vi "CmdExe.Check StdOut, StdError, and Return Code for errors, Merge to Output Data.vi"(6 "Error Check":T1, 7 "App Name":string, 8 "error in":errorcluster, 9 "Return Code":i32, 10 "StdError":string, 11 "StdOut":string) -> (0 "error out":errorcluster, 3 "Output Data":string)   [LabVIEW 2024]
uses:
  CmdExe.Output Error Check Setup.ctl
  Errors/Error.Error Code List.ctl
  <vilib>/Utility/error.llb/Trim Whitespace One-Sided.vi
  Errors.lvlib
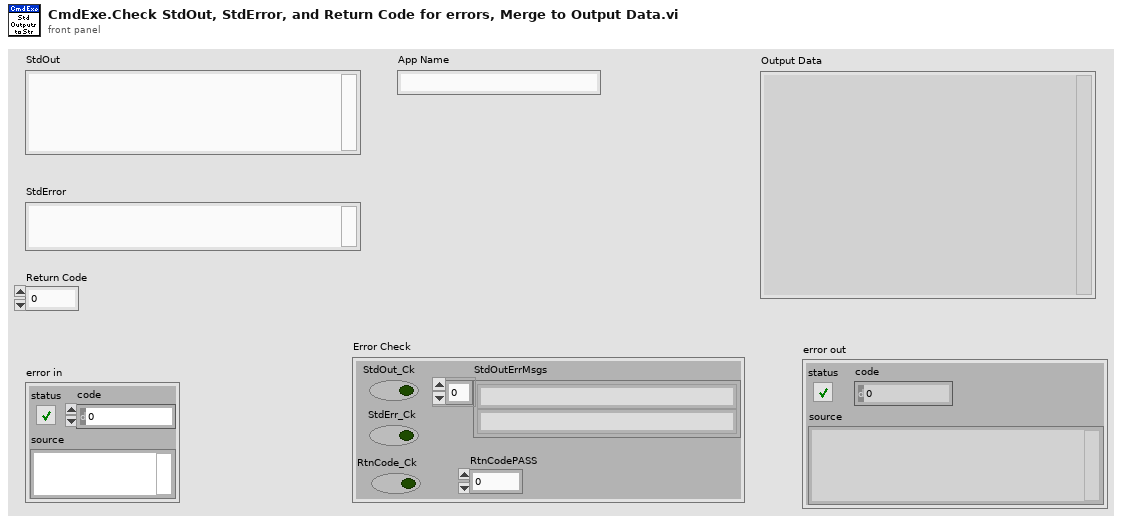
[diagram p1: front panel]
types:
  T1 = typedef "CmdExe.Output Error Check Setup.ctl" = cluster{"StdOut_Ck":bool, "StdOutErrMsgs":string[], "StdErr_Ck":bool, "RtnCode_Ck":bool, "RtnCodePASS":i32}
  T2 = typedef "EQMF.lvlib/Errors.lvlib/Error.Error Code List.ctl" = i32
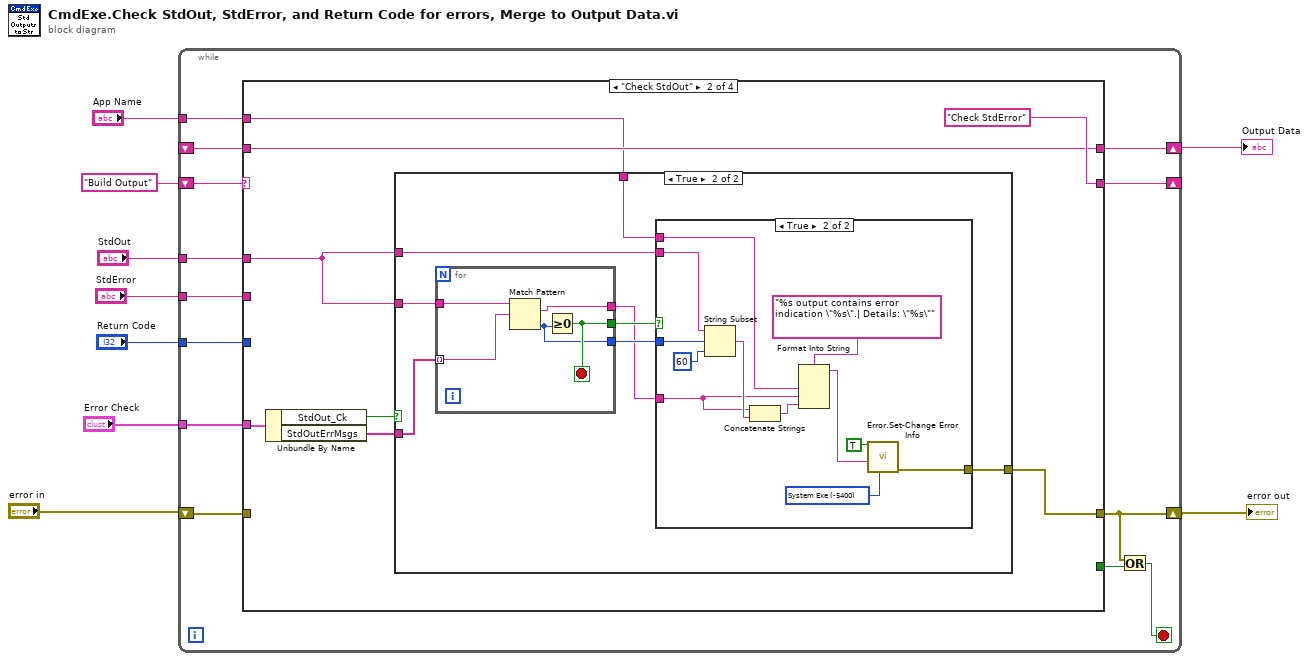
[diagram p0: block diagram]
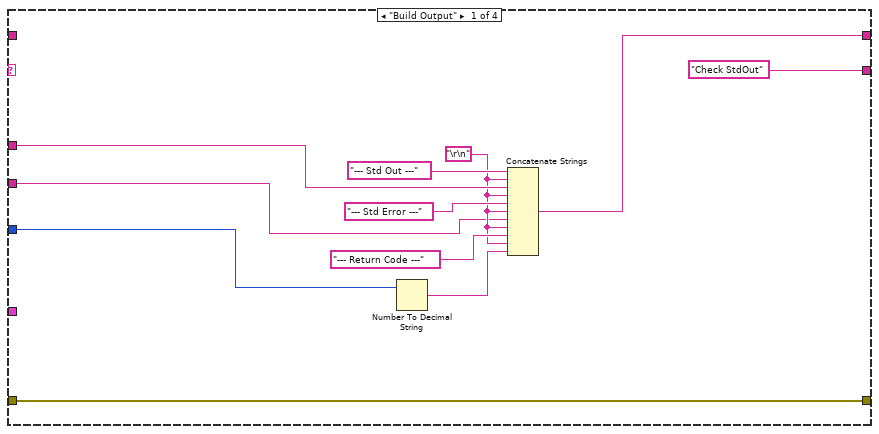
[diagram p2: hidden frame]
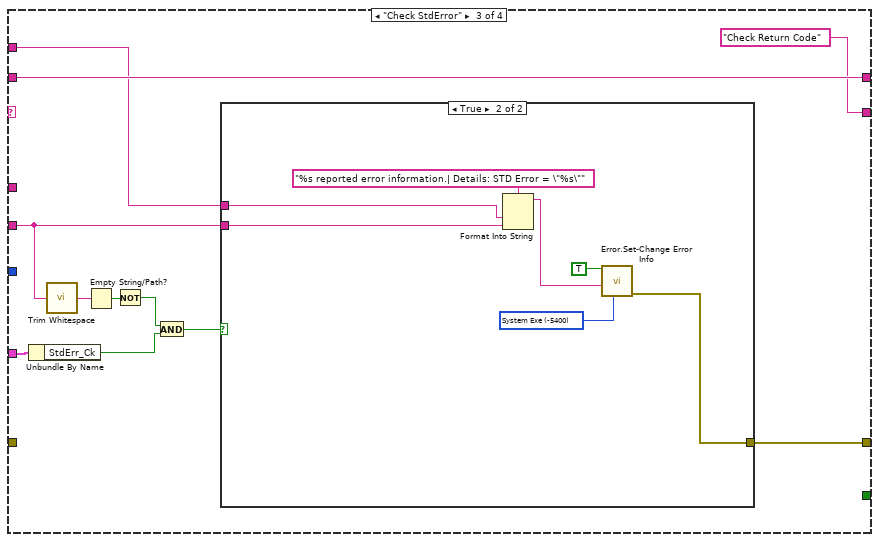
[diagram p5: hidden frame]
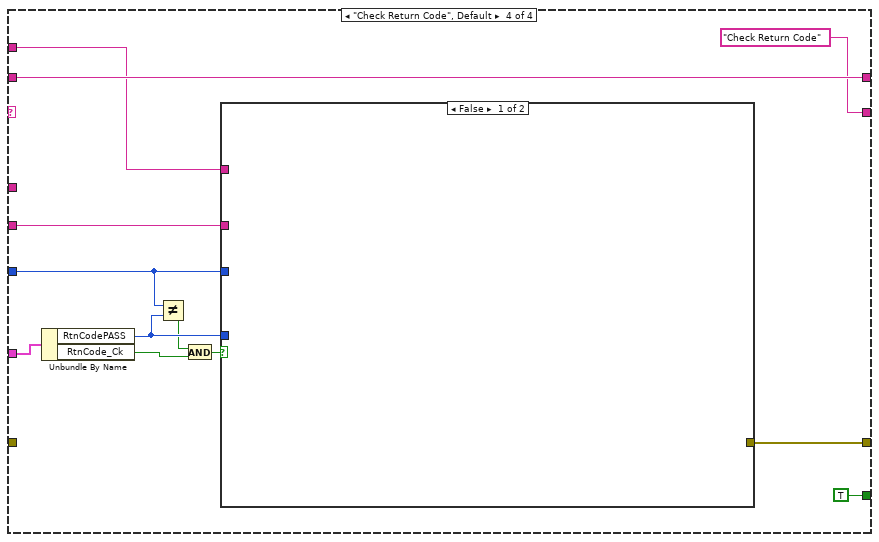
[diagram p7: hidden frame]
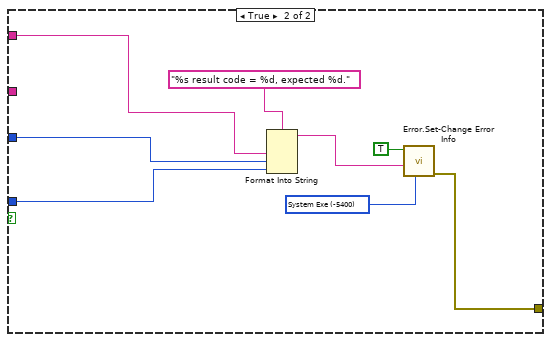
[diagram p8: hidden frame]
diagram:
  n1 = while {
    shift-right: [w17] -> _
    shift-left: "Build Output" -> [w22]
    tunnel: "Error Check" -> [w21]
    tunnel: "StdOut" -> [w20]
    tunnel: "StdError" -> [w19]
    tunnel: "Return Code" -> [w18]
    shift-right: [w16] -> w4
    shift-left: _ -> [w15]
    shift-right: [w13] -> w3
    shift-left: "error in" -> [w14]
    tunnel: "App Name" -> [w10]
    stop <- w11 stop-if-true
    n2 = case shown="\"Check StdOut\"" w22 {
      tunnel: w21 -> [_ w39 w71 w92]
      tunnel: w20 -> [w32 w36 _ _]
      tunnel: w19 -> [w23 _ w73 w93]
      tunnel: w18 -> [w28 _ _ w90]
      tunnel: ["Check StdOut" "Check StdError" "Check Return Code" "Check Return Code"] -> w17
      tunnel: [w26 w40 w77 w96] -> w16
      tunnel: w15 -> [_ w40 w77 w96]
      tunnel: [w25 w35 w75 w94] -> w13
      tunnel: w14 -> [w25 _ _ _]
      tunnel: [_ _ _ TRUE] -> w12
      tunnel: w10 -> [_ w34 w67 w85]
      frame "Build Output" {
        w24 = "\r\n"
        n3 = Number To Decimal String(number=w28) -> (decimal integer string=w29:string)  [unwired: 1 in]
        n4 = Concatenate Strings("--- Std Out ---", w24, w32, w24, "--- Std Error ---", w24, w23, w24, "--- Return Code ---", w24, w29) -> (w26:string)
      }
      frame "Check StdOut" {
        n5 = Unbundle By Name(w39) -> ("StdOut_Ck"=w38:bool, "StdOutErrMsgs"=w37:string[])
        n6 = case shown="True" w38 {
          tunnel: w37 -> [_ w48]
          tunnel: w36 -> [_ w49]
          tunnel: w36 -> [_ w45]
          tunnel: [_ w44] -> w35
          tunnel: w34 -> [_ w42]
          frame False {
          }
          frame True {
            n7 = for {
              tunnel: w49 -> [w66]
              tunnel: [w63] -> w43
              tunnel: [w65] -> w47
              tunnel: w48 -> [w62] mode=indexing
              tunnel: [w64] -> w46
              stop <- w65 stop-if-true
              n8 = Match Pattern(string=w66, regular expression=w62) -> (match substring=w63:string, offset past match=w64:i32)  [unwired: 1 in, 2 out]
              n9 = Greater Or Equal To 0?(x=w64) -> (x >= 0?=w65:bool)
            }
            n10 = case shown="True" w47 {
              tunnel: w43 -> [_ w51]
              tunnel: [_ w57] -> w44
              tunnel: w46 -> [_ w56]
              tunnel: w45 -> [_ w54]
              tunnel: w42 -> [_ w50]
              frame False {
              }
              frame True {
                w59 = T2 -5400 items=["No Error"=0, "Abort"=-2, "Misc"=-5000, "Fixture Error"=-5100, "File IO - General"=-5200, "FIle IO - Config Error"=-5201, "Instrument - General"=-5300, "Instrument - Serial Com"=-5301, "Instrument - Camera"=-5302, "Instrument - PS"=-5303, "Instrument - Oscilloscope"=-5304, "Instrument - Function Gen"=-5305, "Instrument - Load"=-5306, "Instrument - Meter"=-5307, "Instrument - Power Control"=-5308, "Instrument - Motion"=-5309, "Instrument - RF"=-5310, "System Exe"=-5400, "Image Processing"=-5500, "Communication"=-5600, "Script - Syntax Error"=-6000, "Script - Invalid Name or Param"=-6100, "Script - Timeout"=-6200, "Invalid Data"=-6300] ("Std Code")
                n11 = String Subset(string=w54, offset (0)=w56, length (rest)=60 ("length (rest)")) -> (substring=w52:string)
                n12 = Concatenate Strings(w51, w52) -> (w53:string)
                n13 = Format Into String(format string="%s output contains error indication \"%s\".| Details: \"%s\"", w50, w51, w53) -> (resulting string=w58:string)  [unwired: 2 in, 1 out]
                n14 = call "Error.Set-Change Error Info.vi"("Std Code"=w59, "Description"=w58, "Set Error"=TRUE) -> ("error out"=w57:errorcluster)  [unwired: 8 in]
              }
            }
          }
        }
      }
      frame "Check StdError" {
        n15 = Unbundle By Name(w71) -> ("StdErr_Ck"=w69:bool)
        n16 = call <vilib>:"Trim Whitespace.vi"("string"=w73) -> ("trimmed string"=w74:string)  [unwired: 1 in]
        n17 = Empty String/Path?(string/path=w74) -> (empty?=w72:bool)
        n18 = Not(x=w72) -> (.not. x?=w70:bool)
        n19 = And(x=w70, y=w69) -> (x .and. y?=w68:bool)
        n20 = case shown="True" w68 {
          tunnel: w73 -> [_ w80]
          tunnel: [_ w79] -> w75
          tunnel: w67 -> [_ w78]
          frame False {
          }
          frame True {
            w82 = T2 -5400 items=["No Error"=0, "Abort"=-2, "Misc"=-5000, "Fixture Error"=-5100, "File IO - General"=-5200, "FIle IO - Config Error"=-5201, "Instrument - General"=-5300, "Instrument - Serial Com"=-5301, "Instrument - Camera"=-5302, "Instrument - PS"=-5303, "Instrument - Oscilloscope"=-5304, "Instrument - Function Gen"=-5305, "Instrument - Load"=-5306, "Instrument - Meter"=-5307, "Instrument - Power Control"=-5308, "Instrument - Motion"=-5309, "Instrument - RF"=-5310, "System Exe"=-5400, "Image Processing"=-5500, "Communication"=-5600, "Script - Syntax Error"=-6000, "Script - Invalid Name or Param"=-6100, "Script - Timeout"=-6200, "Invalid Data"=-6300] ("Std Code")
            n21 = Format Into String(format string="%s reported error information.| Details: STD Error = \"%s\"", w78, w80) -> (resulting string=w81:string)  [unwired: 2 in, 1 out]
            n22 = call "Error.Set-Change Error Info.vi"("Std Code"=w82, "Description"=w81, "Set Error"=TRUE) -> ("error out"=w79:errorcluster)  [unwired: 8 in]
          }
        }
      }
      frame "Check Return Code", Default {
        n23 = Unbundle By Name(w92) -> ("RtnCodePASS"=w89:i32, "RtnCode_Ck"=w86:bool)
        n24 = Not Equal?(x=w90, y=w89) -> (x != y?=w87:bool)
        n25 = And(x=w87, y=w86) -> (x .and. y?=w88:bool)
        n26 = case shown="False" w88 {
          tunnel: w93 -> [_ _]
          tunnel: [_ w98] -> w94
          tunnel: w90 -> [_ w100]
          tunnel: w89 -> [_ w99]
          tunnel: w85 -> [_ w97]
          frame False {
          }
          frame True {
            w104 = T2 -5400 items=["No Error"=0, "Abort"=-2, "Misc"=-5000, "Fixture Error"=-5100, "File IO - General"=-5200, "FIle IO - Config Error"=-5201, "Instrument - General"=-5300, "Instrument - Serial Com"=-5301, "Instrument - Camera"=-5302, "Instrument - PS"=-5303, "Instrument - Oscilloscope"=-5304, "Instrument - Function Gen"=-5305, "Instrument - Load"=-5306, "Instrument - Meter"=-5307, "Instrument - Power Control"=-5308, "Instrument - Motion"=-5309, "Instrument - RF"=-5310, "System Exe"=-5400, "Image Processing"=-5500, "Communication"=-5600, "Script - Syntax Error"=-6000, "Script - Invalid Name or Param"=-6100, "Script - Timeout"=-6200, "Invalid Data"=-6300] ("Std Code")
            n27 = Format Into String(format string="%s result code = %d, expected %d.", w97, w100, w99) -> (resulting string=w101:string)  [unwired: 2 in, 1 out]
            n28 = call "Error.Set-Change Error Info.vi"("Std Code"=w104, "Description"=w101, "Set Error"=TRUE) -> ("error out"=w98:errorcluster)  [unwired: 8 in]
          }
        }
      }
    }
    n29 = Or(x=w13, y=w12) -> (x .or. y?=w11:bool)
  }
  "error out" <- w3
  "Output Data" <- w4
